vi "Cleanup.vi"(8 "error in (no error)":errorcluster) -> (0 "error out":errorcluster)   [LabVIEW 2011]
uses:
  030 - EVENTS/03 - ToMessageHandlerProcess/enumMessageCriticity.ctl
  090 - ERRORS/Ctrls/enumLogAndView.ctl
  030 - EVENTS/EnumFgvEventCommand.ctl
  100_PROCESS/SubVis/EnumFgvReferenceProcess.ctl
  090 - ERRORS/Ctrls/EnumErrors.ctl
  080 - TOOLS/Traduction/Dictionnary/EnumCommandDictionnaire.ctl
panel:
  # "CLEANUP"
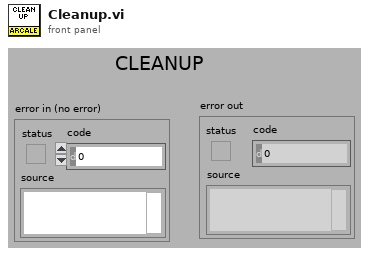
[diagram p1: front panel]
types:
  T1 = typedef "enumMessageCriticity.ctl" = enum16{"No error", "Info", "Warning", "Error", "Fatal error"}
  T2 = typedef "enumLogAndView.ctl" = enum16{"Log only", "Log and view"}
  T3 = typedef "EnumFgvEventCommand.ctl" = enum16{"Setup", "Cleanup", "Get"}
  T4 = typedef "EnumFgvReferenceProcess.ctl" = enum16{"Init", "Get", "Add Reference", "Close References"}
  T5 = typedef "EnumErrors.ctl" = enum16{"VI non trouvé !", "Clé non trouvée", "Timeout", "Le VI tourne déjà", "Erreur de séparateur décimal", "Référence non trouvée"}
  T6 = typedef "EnumCommandDictionnaire.ctl" = enum16{"Load", "Translate", "Save", "GetDico", "Set : A traduire = Vrai", "Set : A Traduire = Faux", "SetDico"}
  T7 = typedef "FromProcessesEventType.ctl" = enum16{"Started", "Autotest", "Ended"}
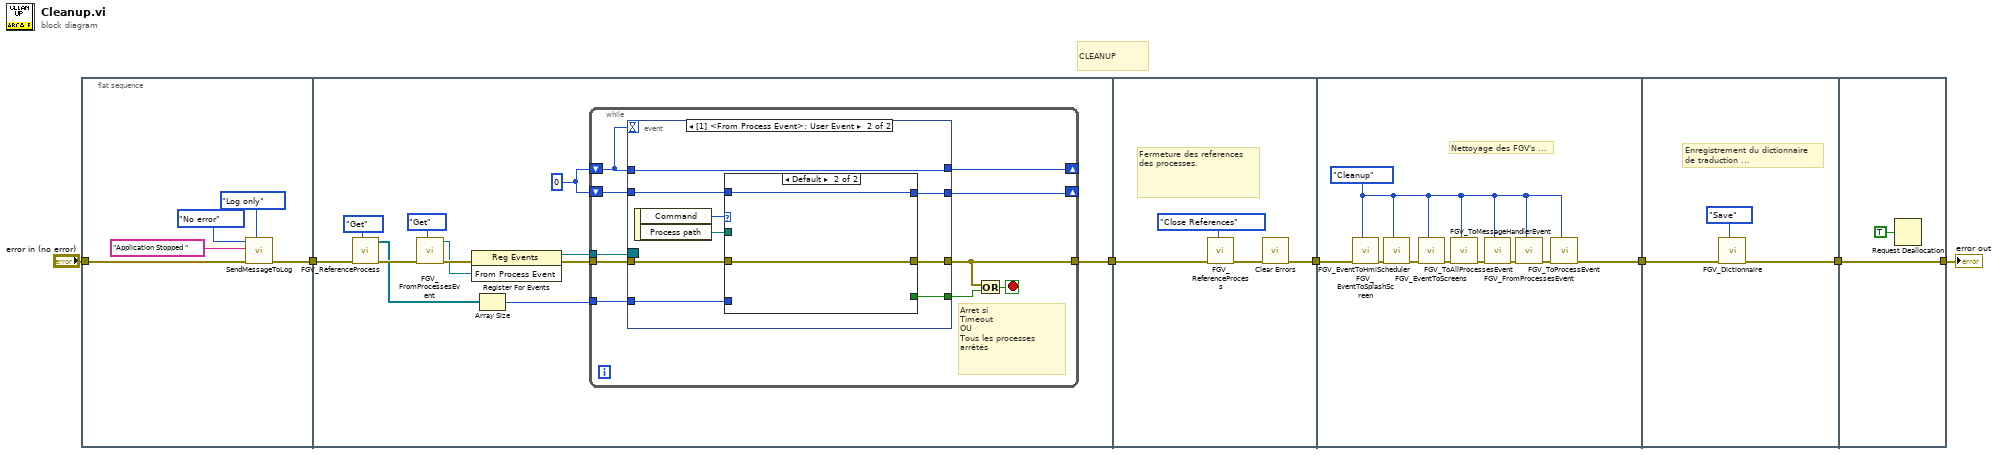
[diagram p0: block diagram]
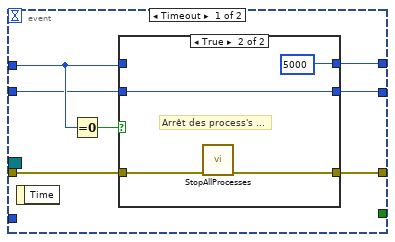
[diagram p2: hidden frame]
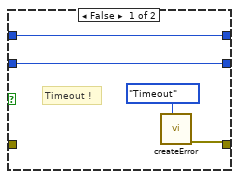
[diagram p3: hidden frame]
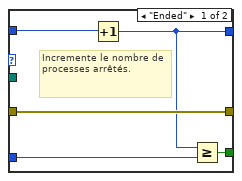
[diagram p4: hidden frame]
diagram:
  # "CLEANUP"
  n1 = flat-sequence {
    tunnel: "error in (no error)" -> [w9]
    tunnel: [w8] -> w5
    tunnel: [w24] -> w3
    tunnel: w5 -> [w23]
    tunnel: w3 -> [w69]
    tunnel: [w66] -> w2
    tunnel: [w71] -> w4
    tunnel: w2 -> [w78]
    tunnel: w4 -> [w81]
    tunnel: [w80] -> w1
    tunnel: [w83] -> w6
    tunnel: w1 -> [w83]
    frame #0 {
      n2 = call "SendMessageToLog.vi"("Log and view ?"=enumLogAndView."Log only", "error in (no error)"=w9, "Message"="Application Stopped ", "Criticity"=enumMessageCriticity."No error") -> ("error out"=w8:errorcluster)  [unwired: 7 in]
    }
    frame #1 {
      w13 = 0
      n3 = call "FGV_ReferenceProcess.vi"("Commande"=EnumFgvReferenceProcess."Get", "error in (no error)"=w23) -> ("error out"=w21:errorcluster, "ProcessReferences"=w15:refnum<vi>[])  [unwired: 8 in]
      n4 = call "FGV_FromProcessesEvent.vi"("Command"=EnumFgvEventCommand."Get", "error in (no error)"=w21) -> ("error out"=w19:errorcluster, "From Process Event"=w17:refnum<user-event>)  [unwired: 8 in]
      n5 = register-events(error in=w19, w17) -> (reference out=w16:refnum<event-registration>, error out=w18:errorcluster)  [unwired: 1 in]
      n6 = Array Size(array=w15) -> (size(s)=w14:i32)
      n7 = while {
        tunnel: [w25] -> w24
        tunnel: w18 -> [w34]
        tunnel: w16 -> [w33]
        shift-right: [w32] -> _
        shift-left: w13 -> [w31]
        tunnel: w14 -> [w30]
        shift-right: [w27] -> _
        shift-left: w13 -> [w28]
        stop <- w29 stop-if-true
        # "Arret si \nTimeout\nOU\nTous les processes arrêtés"
        n8 = event shown="[1] <From Process Event>: User Event" {
          selector: w33 -> [_ _]
          dyn-events: _ -> [_ _]
          timeout: w31 -> [_ _]
          tunnel: [w41 w57] -> w25
          tunnel: w34 -> [w40 w58]
          tunnel: w31 -> [w37 w50]
          tunnel: [w38 w50] -> w32
          tunnel: w30 -> [_ w52]
          tunnel: w28 -> [w36 w54]
          tunnel: [w35 w53] -> w27
          tunnel: [_ w51] -> w26
          event Timeout {
            n9 = event-data() -> ()  [unwired: 1 in, 1 out]
            n10 = Equal To 0?(x=w37) -> (x = 0?=w39:bool)
            n11 = case shown="True" w39 {
              tunnel: [w42 w49] -> w41
              tunnel: w40 -> [_ w48]
              tunnel: [w45 5000] -> w38
              tunnel: w37 -> [w45 _]
              tunnel: w36 -> [w44 w46]
              tunnel: [w44 w46] -> w35
              frame False {
                # "Timeout !"
                n12 = call "createError.vi"("ErrorCode"=EnumErrors."Timeout") -> ("error out"=w42:errorcluster)  [unwired: 10 in]
              }
              frame True {
                # "Arrêt des process's ..."
                n13 = call "StopAllProcesses.vi"("error in (no error)"=w48) -> ("error out"=w49:errorcluster)  [unwired: 10 in]
              }
            }
          }
          event User Event {
            n14 = event-data() -> ("Command"=w56:T7, "Process path"=w55:path)  [unwired: 1 in]
            n15 = case shown="Default" w56 {
              tunnel: w58 -> [w63 w65]
              tunnel: [w63 w65] -> w57
              tunnel: w55 -> [_ _]
              tunnel: w54 -> [w62 w64]
              tunnel: [w61 w64] -> w53
              tunnel: w52 -> [w60 _]
              tunnel: [w59 _] -> w51
              frame "Ended" {
                # "Incremente le nombre de processes arrêtés."
                n16 = Increment(x=w62) -> (x+1=w61:i32)
                n17 = Greater Or Equal?(x=w61, y=w60) -> (x >= y?=w59:bool)
              }
              frame Default {
              }
            }
          }
        }
        n18 = Or(x=w25, y=w26) -> (x .or. y?=w29:bool)
      }
    }
    frame #2 {
      # "Fermeture des references des processes."
      n19 = call "FGV_ReferenceProcess.vi"("Commande"=EnumFgvReferenceProcess."Close References", "error in (no error)"=w69) -> ("error out"=w67:errorcluster)  [unwired: 8 in, 1 out]
      n20 = call <vilib>:"Clear Errors.vi"("error in (no error)"=w67) -> ("error out"=w66:errorcluster)  [unwired: 6 in]
    }
    frame #3 {
      w70 = EnumFgvEventCommand."Cleanup" ("Command")
      # "Nettoyage des FGV's ..."
      n21 = call "FGV_EventToSplashScreen.vi"("Command"=w70, "error in (no error)"=w78) -> ("error out"=w77:errorcluster)  [unwired: 8 in, 1 out]
      n22 = call "FGV_EventToHmiScheduler.vi"("Command"=w70, "error in (no error)"=w77) -> ("error out"=w76:errorcluster)  [unwired: 8 in, 1 out]
      n23 = call "FGV_EventToScreens.vi"("Command"=w70, "error in (no error)"=w76) -> ("error out"=w75:errorcluster)  [unwired: 8 in, 1 out]
      n24 = call "FGV_ToMessageHandlerEvent.vi"("Command"=w70, "error in (no error)"=w75) -> ("error out"=w74:errorcluster)  [unwired: 8 in, 1 out]
      n25 = call "FGV_ToAllProcessesEvent.vi"("Command"=w70, "error in (no error)"=w74) -> ("error out"=w73:errorcluster)  [unwired: 8 in, 1 out]
      n26 = call "FGV_FromProcessesEvent.vi"("Command"=w70, "error in (no error)"=w73) -> ("error out"=w72:errorcluster)  [unwired: 8 in, 1 out]
      n27 = call "FGV_ToProcessEvent.vi"("Command"=w70, "error in (no error)"=w72) -> ("error out"=w71:errorcluster)  [unwired: 8 in, 1 out]
    }
    frame #4 {
      # "Enregistrement du dictionnaire\nde traduction ..."
      n28 = call "FGV_Dictionnaire.vi"("Command"=EnumCommandDictionnaire."Save", "error in (no error)"=w81) -> ("error out"=w80:errorcluster)  [unwired: 7 in, 2 out]
    }
    frame #5 {
      n29 = Request Deallocation(TRUE ("flag")) -> ()
    }
  }
  "error out" <- w6
